vi "Message Loop Error Status.vi"(9 "Message":refnum<class "Client Message.lvclass">, 11 "OBS in":refnum<class "OBS.lvclass">) -> (0 "error out":errorcluster, 3 "OBS out":refnum<class "OBS.lvclass">)   [LabVIEW 2022 SP3, in "obs-websocket-lv.lvlib" / "OBS.lvclass"]
uses:
  OBS.lvclass
  OBS.lvclass/OBS.ctl
  Identify/Identify.lvclass
  Client Message/Client Message.lvclass
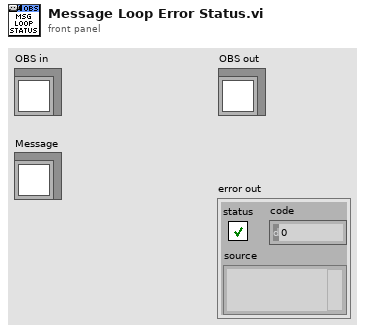
[diagram p1: front panel]
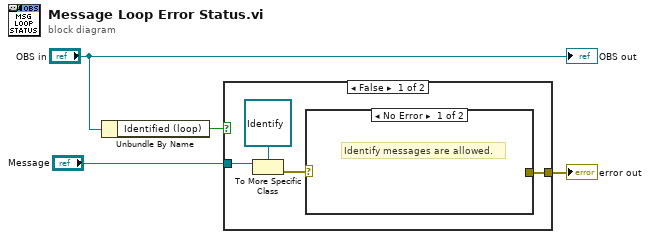
[diagram p0: block diagram]
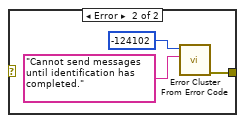
[diagram p2: hidden frame]
diagram:
  n1 = Unbundle By Name("OBS in") -> ("Identified (loop)"=w3:bool)
  n2 = case shown="False" w3 {
    tunnel: "Message" -> [w8 _]
    tunnel: [w5 _] -> w1
    frame False {
      n3 = To More Specific Class(target class=refnum<class "Identify.lvclass"> refnum ("obs-websocket-lv.lvlib:Identify.lvclass"), reference=w8) -> (error out=w6:errorcluster)  [unwired: 1 in, 1 out]
      n4 = case shown="No Error" w6 {
        tunnel: [_ w11] -> w5
        frame No Error {
          # "Identify messages are allowed."
        }
        frame Error {
          n5 = call <vilib>:"Error Cluster From Error Code.vi"("error message (\"\")"="Cannot send messages until identification has completed." ("error message (\"\")"), "error code (0)"=-124102) -> ("error out"=w11:errorcluster)  [unwired: 7 in]
        }
      }
    }
    frame True {
    }
  }
  "error out" <- w1
  "OBS out" <- "OBS in"
